vi "Flow Sensors Control_beta.vi"(10 "Numeric in":i32, 11 "Cluster in":T1) -> (1 "Cluster 3":cluster{dbl, dbl, dbl, dbl, dbl}, 2 "Numeric out":i32, 3 "Cluster out":T1)   [LabVIEW 2015]
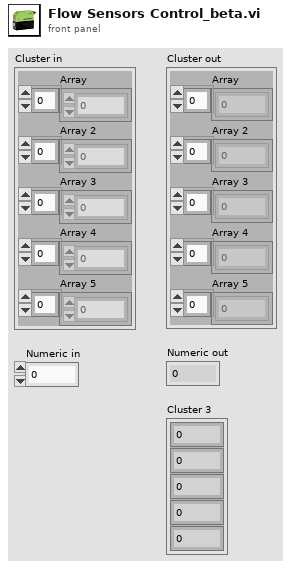
[diagram p1: front panel]
types:
  T1 = cluster{"Array":dbl[], "Array 2":dbl[], "Array 3":dbl[], "Array 4":dbl[], "Array 5":dbl[]}
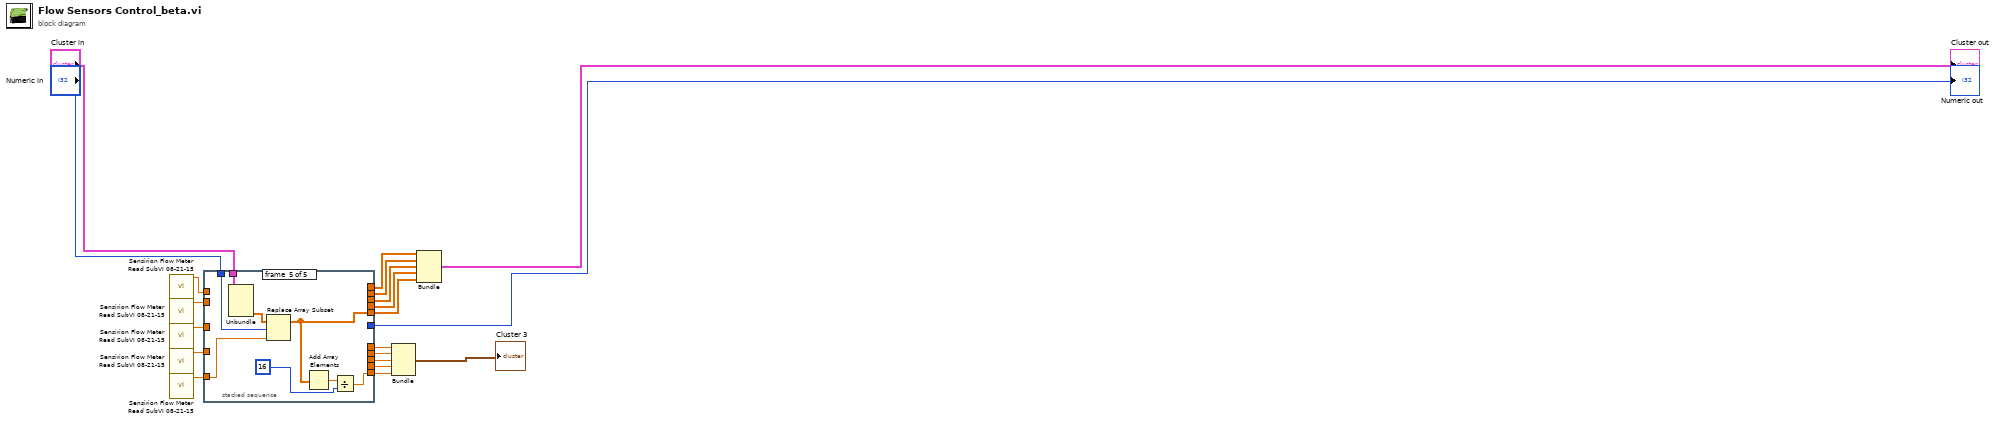
[diagram p0: block diagram]
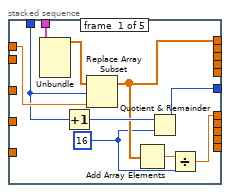
[diagram p2: hidden frame]
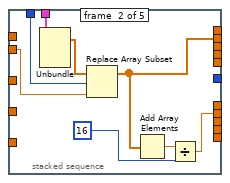
[diagram p3: hidden frame]
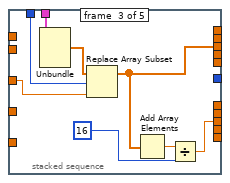
[diagram p4: hidden frame]
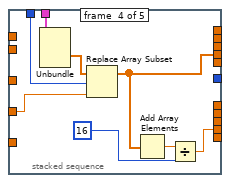
[diagram p5: hidden frame]
diagram:
  n1 = call "Sensirion Flow Meter Read SubVI 08-21-15.vi"() -> ("MeasureResult Scaled"=w2:dbl)  [unwired: 11 in]
  n2 = call "Sensirion Flow Meter Read SubVI 08-21-15.vi"() -> ("MeasureResult Scaled"=w15:dbl)  [unwired: 11 in]
  n3 = call "Sensirion Flow Meter Read SubVI 08-21-15.vi"() -> ("MeasureResult Scaled"=w16:dbl)  [unwired: 11 in]
  n4 = call "Sensirion Flow Meter Read SubVI 08-21-15.vi"() -> ("MeasureResult Scaled"=w17:dbl)  [unwired: 11 in]
  n5 = call "Sensirion Flow Meter Read SubVI 08-21-15.vi"() -> ("MeasureResult Scaled"=w18:dbl)  [unwired: 11 in]
  n6 = stacked-sequence {
    tunnel: [w26 _ _ _ _] -> w4
    tunnel: "Numeric in" -> [w27 w38 w46 w54 w62]
    tunnel: [w29 _ _ _ _] -> w20
    tunnel: w2 -> [w28 _ _ _ _]
    tunnel: [w23 _ _ _ _] -> w3
    tunnel: "Cluster in" -> [w22 w33 w43 w51 w59]
    tunnel: [_ w35 _ _ _] -> w5
    tunnel: [_ w34 _ _ _] -> w6
    tunnel: [_ _ w42 _ _] -> w9
    tunnel: [_ _ w41 _ _] -> w10
    tunnel: [_ _ _ w50 _] -> w11
    tunnel: [_ _ _ w49 _] -> w12
    tunnel: [_ _ _ _ w58] -> w13
    tunnel: [_ _ _ _ w56] -> w14
    tunnel: w15 -> [_ w31 _ _ _]
    tunnel: w16 -> [_ _ w39 _ _]
    tunnel: w17 -> [_ _ _ w47 _]
    tunnel: w18 -> [_ _ _ _ w55]
    frame #0 {
      w24 = 16 ("y")
      n7 = Unbundle(w22) -> ("Array"=w21:dbl[])  [unwired: 4 out]
      n8 = Increment(x=w27) -> (x+1=w30:i32)
      n9 = Replace Array Subset(array=w21, new element=w28, index=w27) -> (w26:dbl[])
      n10 = Add Array Elements(numeric array=w26) -> (sum=w25:dbl)
      n11 = Quotient & Remainder(x=w30, y=w24) -> (x-y*floor(x/y)=w29:i32)  [unwired: 1 out]
      n12 = Divide(x=w25, y=w24) -> (x/y=w23:dbl)
    }
    frame #1 {
      n13 = Unbundle(w33) -> ("Array 2"=w32:dbl[])  [unwired: 4 out]
      n14 = Replace Array Subset(array=w32, new element=w31, index=w38) -> (w34:dbl[])
      n15 = Add Array Elements(numeric array=w34) -> (sum=w37:dbl)
      n16 = Divide(x=w37, y=16) -> (x/y=w35:dbl)
    }
    frame #2 {
      n17 = Unbundle(w43) -> ("Array 3"=w40:dbl[])  [unwired: 4 out]
      n18 = Replace Array Subset(array=w40, new element=w39, index=w46) -> (w41:dbl[])
      n19 = Add Array Elements(numeric array=w41) -> (sum=w45:dbl)
      n20 = Divide(x=w45, y=16) -> (x/y=w42:dbl)
    }
    frame #3 {
      n21 = Unbundle(w51) -> ("Array 4"=w48:dbl[])  [unwired: 4 out]
      n22 = Replace Array Subset(array=w48, new element=w47, index=w54) -> (w50:dbl[])
      n23 = Add Array Elements(numeric array=w50) -> (sum=w53:dbl)
      n24 = Divide(x=w53, y=16) -> (x/y=w49:dbl)
    }
    frame #4 {
      n25 = Unbundle(w59) -> ("Array 5"=w57:dbl[])  [unwired: 4 out]
      n26 = Replace Array Subset(array=w57, new element=w55, index=w62) -> (w58:dbl[])
      n27 = Add Array Elements(numeric array=w58) -> (sum=w61:dbl)
      n28 = Divide(x=w61, y=16) -> (x/y=w56:dbl)
    }
  }
  "Numeric out" <- w20
  n29 = Bundle(w3, w5, w9, w12, w14) -> (→"Cluster 3":cluster{dbl, dbl, dbl, dbl, dbl})  [unwired: 1 in]
  n30 = Bundle("Array"=w4, "Array 2"=w6, "Array 3"=w10, "Array 4"=w11, "Array 5"=w13) -> (→"Cluster out":T1)  [unwired: 1 in]
